vi "Close FIFOs (STM Multi-Client).vi"(8 "error in (no error)":errorcluster, 11 "FIFOs In":T1) -> (0 "error out":errorcluster)   [LabVIEW 2019]
uses:
  FIFOs (STM Multi-Client).ctl
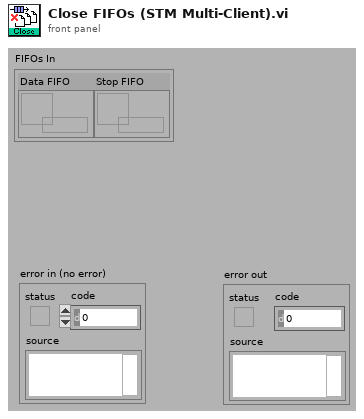
[diagram p1: front panel]
types:
  T1 = typedef "FIFOs (STM Multi-Client).ctl" = cluster{"Data FIFO":refnum<queue>, "Stop FIFO":refnum<queue>}
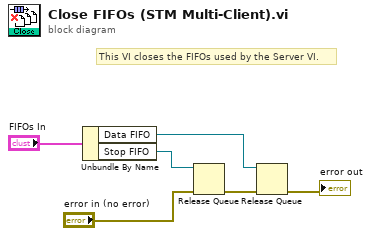
[diagram p0: block diagram]
diagram:
  # "This VI closes the FIFOs used by the Server VI."
  n1 = Unbundle By Name("FIFOs In") -> ("Data FIFO"=w1:refnum<queue>, "Stop FIFO"=w5:refnum<queue>)
  n2 = Release Queue(queue=w5, error in (no error)="error in (no error)") -> (error out=w3:errorcluster)  [unwired: 1 in, 2 out]
  n3 = Release Queue(queue=w1, error in (no error)=w3) -> (error out=→"error out":errorcluster)  [unwired: 1 in, 2 out]
